vi "Key Dialog.vi"(8 "error in":errorcluster, 10 "Key":string, 11 "Config in":refnum<class "Config.lvclass">) -> (0 "error out":errorcluster, 3 "Config out":refnum<class "Config.lvclass">)   [LabVIEW 2023, in "Config.lvlib" / "Config.lvclass"]
uses:
  Config.lvclass
panel:
  out "Dialog":string
  in  "OK Button":bool
  in  "Key Value":string
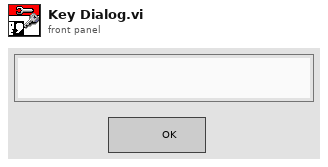
[diagram p1: front panel]
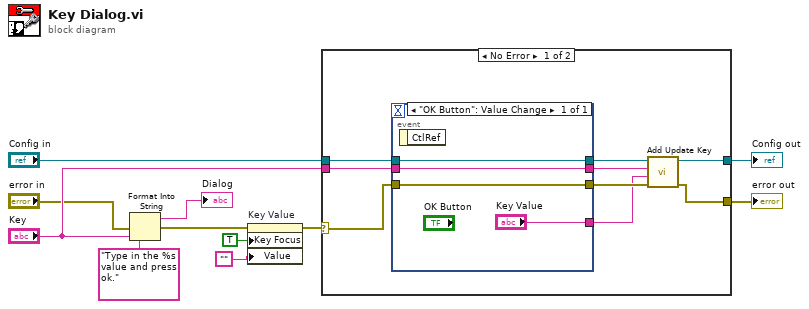
[diagram p0: block diagram]
diagram:
  n1 = Format Into String(format string="Type in the %s value and press ok.", error in="error in", "Key") -> (resulting string=→"Dialog":string, error out=w3:errorcluster)  [unwired: 1 in]
  n2 = property on="Key Value" class="Str"(error in=w3, "Key Focus"=TRUE, "Value"="") -> (error out=w4:errorcluster)  [unwired: 1 in, 1 out]
  n3 = case shown="No Error" w4 {
    selector: w4 -> [w15 w26]
    tunnel: [w19 w26] -> w11
    tunnel: [w20 w25] -> w9
    tunnel: "Config in" -> [w18 w25]
    tunnel: "Key" -> [w13 _]
    frame No Error {
      n4 = event shown="[0] \"OK Button\": Value Change" {
        selector: _ -> [_]
        dyn-events: _ -> [_]
        timeout: _ -> [_]
        tunnel: ["Key Value"] -> w14
        tunnel: w18 -> [w23]
        tunnel: [w23] -> w17
        tunnel: [w22] -> w16
        tunnel: w15 -> [w22]
        tunnel: w13 -> [w21]
        tunnel: [w21] -> w12
        event "OK Button": Value Change {
          n5 = event-data() -> ()  [unwired: 1 in, 1 out]
        }
      }
      n6 = call "Add Update Key.vi"("error in"=w16, "Value"=w14, "Key"=w12, "Config in"=w17) -> ("error out"=w19:errorcluster, "Config out"=w20:refnum<class "Config.lvclass">)  [unwired: 6 in]
    }
    frame Error {
    }
  }
  "error out" <- w11
  "Config out" <- w9
